vi "FGcontrolfor3D211230.vi"(8 "error in (no error)":errorcluster, 9 "query status":bool, 11 "Array 3":T1(array[cluster])) -> (0 "error out":errorcluster={"status"=FALSE, "code"=1073481728, "source"="User Programmed Value out of Range"}, 1 "output":string[](array[string])=["ON", "ON", "ON", "ON"], 2 "burst":T2[](array[typedef])=[{"State"="ON", "Period"="0.030001", "Start Phase"="0", "Trigger Source"="INT", "Trigger Mode"="RISE", "Cycle Time"="3", "Delay"="9.04e-07", "Edge"="", "Gate or N-Cycled"="NCYC", "Polarity"=""}, {"State"="ON", "Period"="", "Start Phase"="", "Trigger Source"="EXT", "Trigger Mode"="", "Cycle Time"="3", "Delay"="9.76e-07", "Edge"="RISE", "Gate or N-Cycled"="NCYC", "Polarity"=""}, {"State"="ON", "Period"="", "Start Phase"="0", "Trigger Source"="EXT", "Trigger Mode"="", "Cycle Time"="3", "Delay"="9.6e-07", "Edge"="RISE", "Gate or N-Cycled"="NCYC", "Polarity"=""}, {"State"="ON", "Period"="", "Start Phase"="", "Trigger Source"="EXT", "Trigger Mode"="", "Cycle Time"="10", "Delay"="3.3e-05", "Edge"="RISE", "Gate or N-Cycled"="NCYC", "Polarity"=""}], 3 "basic":T3[](array[typedef])=[{"Waveform"="RAMP", "Frequency"="100", "Amplitude"="0.01", "Offset"="3", "Phase"="0", "Duty Cycle"="", "Delay"="", "Std Deviation"="", "Mean"="", "Symmetry"="70"}, {"Waveform"="PULSE", "Frequency"="100", "Amplitude"="0.01", "Offset"="3", "Phase"="", "Duty Cycle"="0.1", "Delay"="0", "Std Deviation"="", "Mean"="", "Symmetry"=""}, {"Waveform"="RAMP", "Frequency"="100", "Amplitude"="0.01", "Offset"="4", "Phase"="0", "Duty Cycle"="", "Delay"="", "Std Deviation"="", "Mean"="", "Symmetry"="70"}, {"Waveform"="PULSE", "Frequency"="10000", "Amplitude"="0.0001", "Offset"="3", "Phase"="", "Duty Cycle"="2", "Delay"="0", "Std Deviation"="", "Mean"="", "Symmetry"=""}])   [LabVIEW 2024]
uses:
  old LabVIEW files/labview_Mikami/Teledyne LeCroy WaveStation/Public/Typedefs/Basic Waveform Info.ctl
  old LabVIEW files/labview_Mikami/Teledyne LeCroy WaveStation/Public/Typedefs/Burst Waveform Info.ctl
  old LabVIEW files/labview_Mikami/Teledyne LeCroy WaveStation/Teledyne LeCroy WaveStation.lvlib
panel:
  out "output cluster":cluster{dbl, bool, string}
  out "z":string[](array[string])=["50", "50", "HZ", "HZ"]
  # "FG1 ch2 for galvo img scan"
  # "FG2 ch2 for SCAPE"
  # "FG3 ch1 for AWGtrig"
  # "FG2 ch1 for FG3trig"
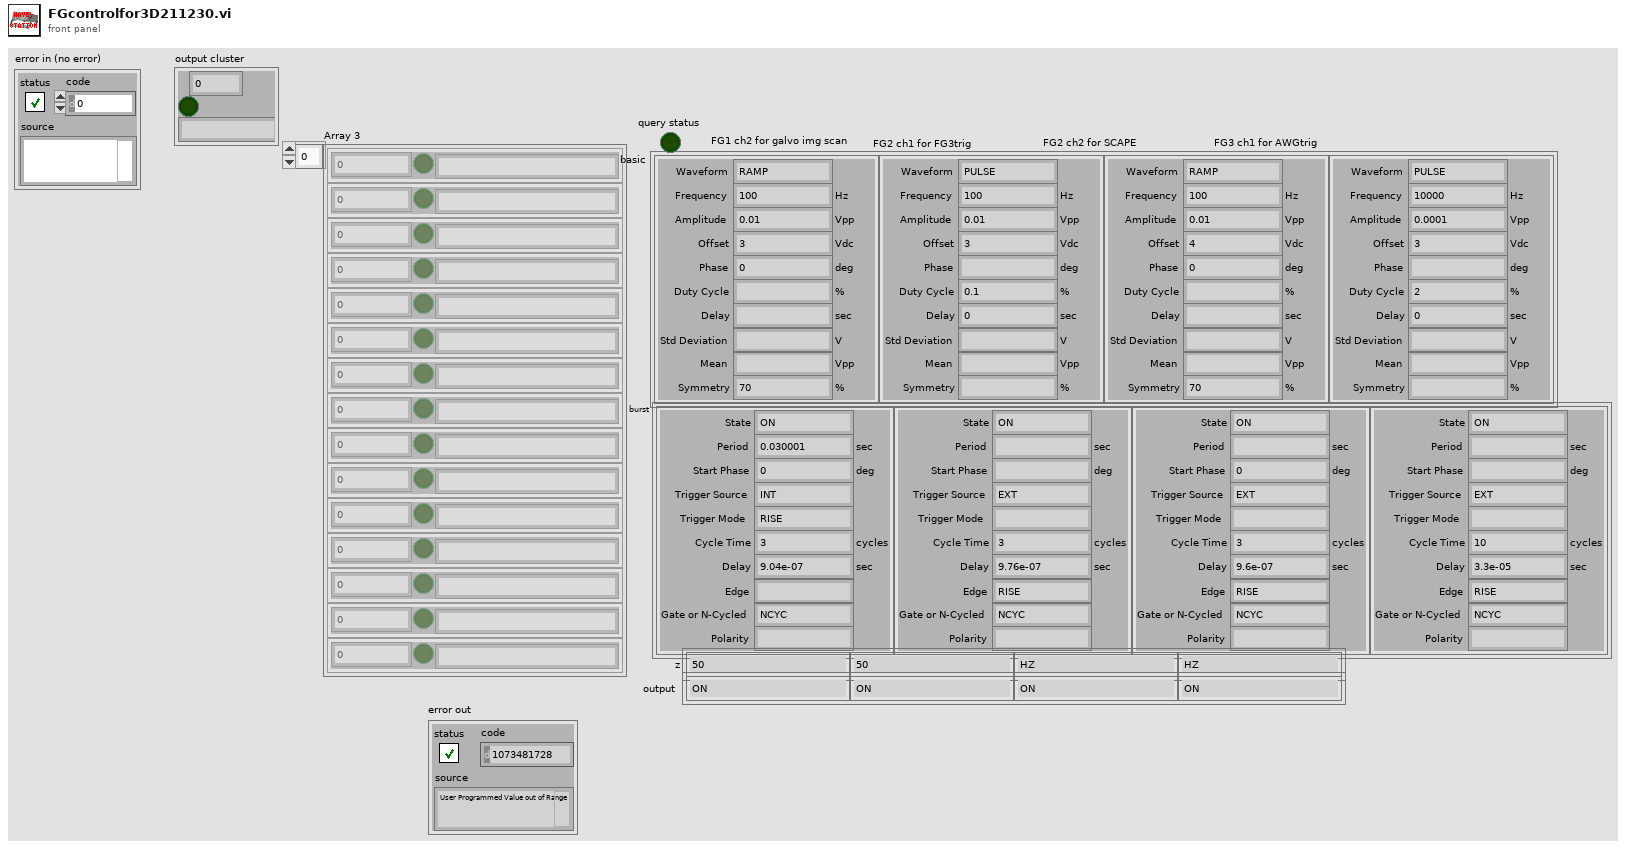
[diagram p1: front panel]
types:
  T1 = cluster{"value":dbl, "on/off":bool, "name":string}[]
  T2 = typedef "Teledyne LeCroy WaveStation.lvlib/Burst Waveform Info.ctl" = cluster{"State":string, "Period":string, "Start Phase":string, "Trigger Source":string, "Trigger Mode":string, "Cycle Time":string, "Delay":string, "Edge":string, "Gate or N-Cycled":string, "Polarity":string}
  T3 = typedef "Teledyne LeCroy WaveStation.lvlib/Basic Waveform Info.ctl" = cluster{"Waveform":string, "Frequency":string, "Amplitude":string, "Offset":string, "Phase":string, "Duty Cycle":string, "Delay":string, "Std Deviation":string, "Mean":string, "Symmetry":string}
  T4 = cluster{"Amplitude (0.004Vpp)":dbl, "ON/OFF":bool, "String":string}
  T5 = cluster{"value":dbl, "on/off":bool, "name":string}
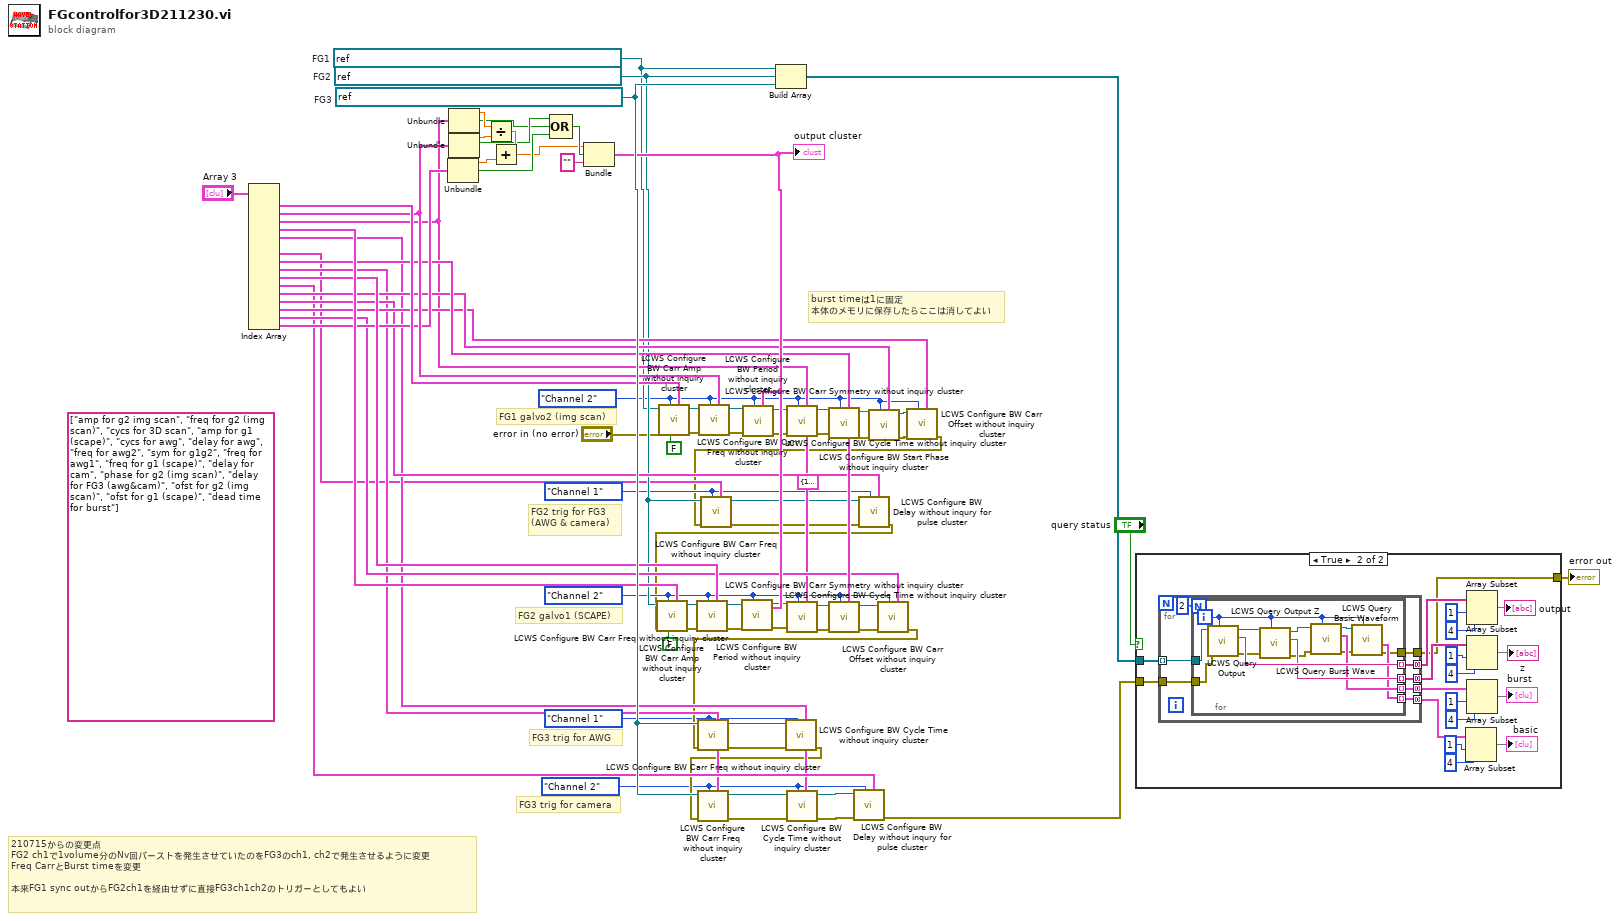
[diagram p0: block diagram]
diagram:
  (unwired) T4 {"Amplitude (0.004Vpp)"=1.0, "ON/OFF"=TRUE, "String"=""} ("input")
  w5 = enum16{"Channel 1", "Channel 2"}."Channel 2" ("Channel (1)")
  w4 = enum16{"Channel 1", "Channel 2"}."Channel 1" ("Channel (1)")
  w24 = enum16{"Channel 1", "Channel 2"}."Channel 1" ("Channel (1)")
  w14 = enum16{"Channel 1", "Channel 2"}."Channel 2" ("Channel (1)")
  w15 = enum16{"Channel 1", "Channel 2"}."Channel 2" ("Channel (1)")
  (unwired) string[] ["amp for g2 img scan", "freq for g2 (img scan)", "cycs for 3D scan", "amp for g1 (scape)", "cycs for awg", "delay for awg", "freq for awg2", "sym for g1g2", "freq for awg1", "freq for g1 (scape)", "delay for cam", "phase for g2 (img scan)", "delay for FG3 (awg&cam)", "ofst for g2 (img scan)", "ofst for g1 (scape)", "dead time for burst"]
  w47 = refnum<visa-resource-name> "USB0::0x05FF::0x0A21::LCRY2362C01698::INSTR"  # FG2
  w72 = refnum<visa-resource-name> "USB0::0x05FF::0x0A21::LCRY2362C01676::INSTR"  # FG3
  w46 = refnum<visa-resource-name> "USB0::0x05FF::0x0A21::LCRY2362C01653::INSTR"  # FG1
  # "burst timeは1に固定\n本体のメモリに保存したらここは消してよい"
  # "FG3 trig for camera"
  # "FG3 trig for AWG"
  # "FG2 galvo1 (SCAPE)"
  # "FG2 trig for FG3 \n(AWG & camera)"
  # "FG1 galvo2 (img scan)"
  # "210715からの変更点\nFG2 ch1で1volume分のNv回バーストを発生させていたのをFG3のch1, ch2で発生させるように変更\nFreq CarrとBurst timeを変更\n\n本来FG1 sync outからFG2ch1を経由せずに直接FG3ch1ch2のトリガーとしてもよい"
  n1 = Index Array(array="Array 3") -> (element #1=w70:T5, element #2=w68:T5, element #3=w48:T5, element #4=w69:T5, element #5=w45:T5, element #7=w43:T5, element #8=w55:T5, element #9=w44:T5, element #10=w65:T5, element #11=w49:T5, element #12=w54:T5, element #13=w51:T5, element #14=w53:T5, element #15=w52:T5, element #16=w63:T5)  [unwired: 16 in, 1 out]
  n2 = Unbundle(w63) -> ("value"=w62:dbl, "on/off"=w61:bool)  [unwired: 1 out]
  n3 = Unbundle(w48) -> ("value"=w64:dbl, "on/off"=w56:bool)  [unwired: 1 out]
  n4 = Unbundle(w68) -> ("value"=w67:dbl, "on/off"=w66:bool)  [unwired: 1 out]
  n5 = Divide(x=w64, y=w67) -> (x/y=w75:dbl)
  n6 = Add(x=w75, y=w62) -> (x+y=w58:dbl)
  n7 = Compound Arithmetic op=OR(w66, w56, w61) -> (w60:bool)
  n8 = Bundle(w58, w60, "") -> (w57:cluster{dbl, bool, string})  [unwired: 1 in]
  "output cluster" <- w57
  n9 = call "LCWS Configure BW Carr Amp without inquiry cluster.vi"("input"=w70, "imp 50(T)/HZ(F)"=FALSE, "Channel (1)"=w15, "error in (no error)"="error in (no error)", "VISA resource name"=w46) -> ("error out"=w39:errorcluster, "VISA resource name out"=w42:refnum<visa-resource-name>)  [unwired: 5 in]
  n10 = call "LCWS Configure BW Carr Freq without inquiry cluster.vi"("input"=w68, "Channel (1)"=w15, "error in (no error)"=w39, "VISA resource name"=w42) -> ("error out"=w38:errorcluster, "VISA resource name out"=w41:refnum<visa-resource-name>)  [unwired: 5 in, 1 out]
  n11 = call "LCWS Configure BW Period without inquiry cluster.vi"("input"=w57, "Channel (1)"=w15, "error in (no error)"=w38, "VISA resource name"=w41) -> ("error out"=w37:errorcluster, "VISA resource name out"=w40:refnum<visa-resource-name>)  [unwired: 6 in]
  n12 = Build Array(w46, w47, w72) -> (w76:refnum<visa-resource-name>[])
  n13 = call "LCWS Configure BW Cycle Time without inquiry cluster.vi"("input"=w48, "Channel (1)"=w15, "error in (no error)"=w37, "VISA resource name"=w40) -> ("error out"=w34:errorcluster, "VISA resource name out"=w33:refnum<visa-resource-name>)  [unwired: 6 in]
  n14 = call "LCWS Configure BW Carr Symmetry without inquiry cluster.vi"("input"=w55, "Channel (1)"=w15, "error in (no error)"=w34, "VISA resource name"=w33) -> ("error out"=w22:errorcluster, "VISA resource name out"=w23:refnum<visa-resource-name>)  [unwired: 6 in]
  n15 = call "LCWS Configure BW Start Phase without inquiry cluster.vi"("input"=w54, "Channel (1)"=w15, "error in (no error)"=w22, "VISA resource name"=w23) -> ("error out"=w20:errorcluster, "VISA resource name out"=w17:refnum<visa-resource-name>)  [unwired: 6 in]
  n16 = call "LCWS Configure BW Carr Offset without inquiry cluster.vi"("input"=w53, "Channel (1)"=w15, "error in (no error)"=w20, "VISA resource name"=w17) -> ("error out"=w21:errorcluster)  [unwired: 6 in, 1 out]
  n17 = call "LCWS Configure BW Carr Freq without inquiry cluster.vi"("input"=w43, "Channel (1)"=w24, "error in (no error)"=w21, "VISA resource name"=w47) -> ("error out"=w2:errorcluster, "VISA resource name out"=w3:refnum<visa-resource-name>)  [unwired: 5 in, 1 out]
  n18 = call "LCWS Configure BW Delay without inqury for pulse cluster.vi"("input"=w51, "Channel (1)"=w24, "error in (no error)"=w2, "VISA resource name"=w3) -> ("error out"=w13:errorcluster)  [unwired: 6 in, 1 out]
  n19 = call "LCWS Configure BW Carr Amp without inquiry cluster.vi"("input"=w69, "imp 50(T)/HZ(F)"=FALSE, "Channel (1)"=w14, "error in (no error)"=w13, "VISA resource name"=w47) -> ("error out"=w36:errorcluster, "VISA resource name out"=w35:refnum<visa-resource-name>)  [unwired: 5 in]
  n20 = call "LCWS Configure BW Carr Freq without inquiry cluster.vi"("input"=w65, "Channel (1)"=w14, "error in (no error)"=w36, "VISA resource name"=w35) -> ("error out"=w26:errorcluster, "VISA resource name out"=w28:refnum<visa-resource-name>)  [unwired: 5 in, 1 out]
  n21 = call "LCWS Configure BW Period without inquiry cluster.vi"("input"=w57, "Channel (1)"=w14, "error in (no error)"=w26, "VISA resource name"=w28) -> ("error out"=w25:errorcluster, "VISA resource name out"=w27:refnum<visa-resource-name>)  [unwired: 6 in]
  n22 = call "LCWS Configure BW Cycle Time without inquiry cluster.vi"("input"=w48, "Channel (1)"=w14, "error in (no error)"=w25, "VISA resource name"=w27) -> ("error out"=w32:errorcluster, "VISA resource name out"=w31:refnum<visa-resource-name>)  [unwired: 6 in]
  n23 = call "LCWS Configure BW Carr Symmetry without inquiry cluster.vi"("input"=w55, "Channel (1)"=w14, "error in (no error)"=w32, "VISA resource name"=w31) -> ("error out"=w19:errorcluster, "VISA resource name out"=w18:refnum<visa-resource-name>)  [unwired: 6 in]
  n24 = call "LCWS Configure BW Carr Offset without inquiry cluster.vi"("input"=w52, "Channel (1)"=w14, "error in (no error)"=w19, "VISA resource name"=w18) -> ("error out"=w16:errorcluster)  [unwired: 6 in, 1 out]
  n25 = call "LCWS Configure BW Carr Freq without inquiry cluster.vi"("input"=w44, "Channel (1)"=w4, "error in (no error)"=w16, "VISA resource name"=w72) -> ("error out"=w11:errorcluster, "VISA resource name out"=w12:refnum<visa-resource-name>)  [unwired: 5 in, 1 out]
  n26 = call "LCWS Configure BW Cycle Time without inquiry cluster.vi"("input"=w45, "Channel (1)"=w4, "error in (no error)"=w11, "VISA resource name"=w12) -> ("error out"=w6:errorcluster)  [unwired: 6 in, 1 out]
  n27 = call "LCWS Configure BW Carr Freq without inquiry cluster.vi"("input"=w44, "Channel (1)"=w5, "error in (no error)"=w6, "VISA resource name"=w72) -> ("error out"=w9:errorcluster, "VISA resource name out"=w10:refnum<visa-resource-name>)  [unwired: 5 in, 1 out]
  n28 = call "LCWS Configure BW Cycle Time without inquiry cluster.vi"("input"=w45, "Channel (1)"=w5, "error in (no error)"=w9, "VISA resource name"=w10) -> ("error out"=w7:errorcluster, "VISA resource name out"=w8:refnum<visa-resource-name>)  [unwired: 6 in]
  n29 = call "LCWS Configure BW Delay without inqury for pulse cluster.vi"("input"=w49, "Channel (1)"=w5, "error in (no error)"=w7, "VISA resource name"=w8) -> ("error out"=w50:errorcluster)  [unwired: 6 in, 1 out]
  n30 = case shown="True" "query status" {
    tunnel: w76 -> [_ w96]
    tunnel: w50 -> [w77 w79]
    tunnel: [w77 w78] -> w73
    frame False {
    }
    frame True {
      n31 = for {
        tunnel: w96 -> [w103] mode=indexing
        tunnel: [w102] -> w94 mode=concatenating
        tunnel: [w101] -> w85 mode=concatenating
        tunnel: [w100] -> w83 mode=concatenating
        tunnel: [w99] -> w81 mode=concatenating
        tunnel: w79 -> [w98]
        tunnel: [w97] -> w78
        n32 = for {
          N: 2 -> [_]
          tunnel: w103 -> [w117]
          tunnel: [w113] -> w102 mode=indexing
          tunnel: [w112] -> w101 mode=indexing
          tunnel: [w111] -> w100 mode=indexing
          tunnel: [w110] -> w99 mode=indexing
          tunnel: w98 -> [w109]
          tunnel: [w105] -> w97
          i -> [w118]
          n33 = call "LCWS Query Output.vi"("Channel (1)"=w118, "error in (no error)"=w109, "VISA resource name"=w117) -> ("error out"=w108:errorcluster, "Channel Output Status"=w113:string, "VISA resource name out"=w116:refnum<visa-resource-name>)  [unwired: 6 in]
          n34 = call "LCWS Query Output Z.vi"("Channel (1)"=w118, "error in (no error)"=w108, "VISA resource name"=w116) -> ("error out"=w107:errorcluster, "Output Impedance"=w112:string, "VISA resource name out"=w115:refnum<visa-resource-name>)  [unwired: 6 in]
          n35 = call "LCWS Query Burst Wave.vi"("Channel (1)"=w118, "error in (no error)"=w107, "VISA resource name"=w115) -> ("error out"=w106:errorcluster, "Burst Waveform Information"=w111:T2, "VISA resource name out"=w114:refnum<visa-resource-name>)  [unwired: 6 in]
          n36 = call "LCWS Query Basic Waveform.vi"("Channel (1)"=w118, "error in (no error)"=w106, "VISA resource name"=w114) -> ("error out"=w105:errorcluster, "Basic Waveform Information"=w110:T3)  [unwired: 5 in, 2 out]
        }
      }
      n37 = Array Subset(array=w81, index=1, length=4) -> (→"basic":T3[])
      n38 = Array Subset(array=w94, index=1, length=4) -> (→"output":string[])
      n39 = Array Subset(array=w85, index=1, length=4) -> (→"z":string[])
      n40 = Array Subset(array=w83, index=1, length=4) -> (→"burst":T2[])
    }
  }
  "error out" <- w73
